vi "Create HSL Mask.vi"(11 "Cropped Image":T1) -> (3 "Image Mask":T1)   [LabVIEW 2012]
uses:
  <vilib>/vision/Image Controls.llb/IMAQ Image.ctl
  <vilib>/vision/NI_Vision_Development_Module.lvlib
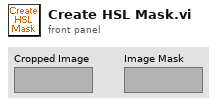
[diagram p1: front panel]
types:
  T1 = typedef "IMAQ Image.ctl" = refnum<image>
  T2 = typedef "Image Type" = u32
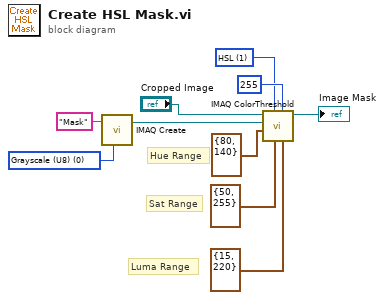
[diagram p0: block diagram]
diagram:
  w5 = u16 1 items=["RGB", "HSL", "HSV", "HSI"] ("Color Mode")
  w2 = T2 0 items=["Grayscale (U8)", "Grayscale (I16)", "Grayscale (SGL)", "Complex (CSG)", "RGB (U32)", "HSL (U32)", "RGB (U64)", "Grayscale (U16)"] ("Image Type")
  # "Luma Range"
  # "Sat Range"
  # "Hue Range"
  n1 = call "IMAQ Create"("Image Name"="Mask", "Image Type"=w2) -> ("New Image"=w4:T1)  [unwired: 3 in, 1 out]
  n2 = call "IMAQ ColorThreshold"("Blue or Luma or Val or Inten Range"=cluster{"Lower value":i32, "Upper value":i32} {"Lower value"=15, "Upper value"=220} ("Luma Range"), "Replace Value"=255, "Green or Sat Range"=cluster{"Lower value":i32, "Upper value":i32} {"Lower value"=50, "Upper value"=255} ("Sat Range"), "Color Mode"=w5, "Red or Hue Range"=cluster{"Lower value":i32, "Upper value":i32} {"Lower value"=80, "Upper value"=140} ("Hue Range"), "Image Dst"=w4, "Image Src"="Cropped Image") -> ("Image Dst Out"=→"Image Mask":T1)  [unwired: 3 in, 1 out]
